vi "Read Nested Count.vi"(11 "Actor with Nesteds in":refnum<class "Actor with Nesteds.lvclass">) -> (2 "Count":i32)   [LabVIEW 2020, in "Actor with Nesteds.lvlib" / "Actor with Nesteds.lvclass"]
uses:
  Actor with Nesteds.lvclass
  Actor with Nesteds.lvclass/Actor with Nesteds.ctl
  ActorFramework/Actor/Actor.lvclass
  C:/justACS/Actor Framework/Core/ActorFramework/Actor/Actor.lvclass
  C:/justACS/Actor Framework/Core/Testing/Test Harness/Actor with Nesteds/Actor with Nesteds/Actor with Nesteds.lvclass
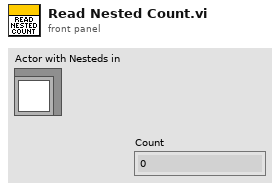
[diagram p1: front panel]
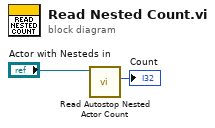
[diagram p0: block diagram]
diagram:
  n1 = call "Read Autostop Nested Actor Count.vi"("Actor in"="Actor with Nesteds in") -> ("Count"=→"Count":i32)  [unwired: 10 in]
